vi "Sent.vi"(8 "error in (no error)":errorcluster, 11 "Mail in":refnum<class "Mail.lvclass">) -> (0 "error out":errorcluster, 3 "Mail out":refnum<class "Mail.lvclass">)   [LabVIEW 2023, in "HardwareAbstractionLayer_LVOOP.lvlib" / "Mail.lvclass"]
uses:
  Mail.lvclass
  Mail.lvclass/Mail.ctl
  <vilib>/smtpClient/LabVIEWSMTPClient.lvlib
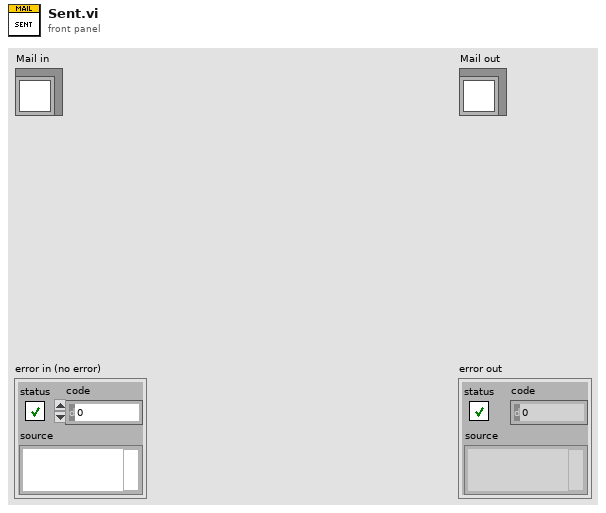
[diagram p1: front panel]
types:
  T1 = typedef "LabVIEWSMTPClient.lvlib/SmtpClientHandle.ctl" = refnum<k1>
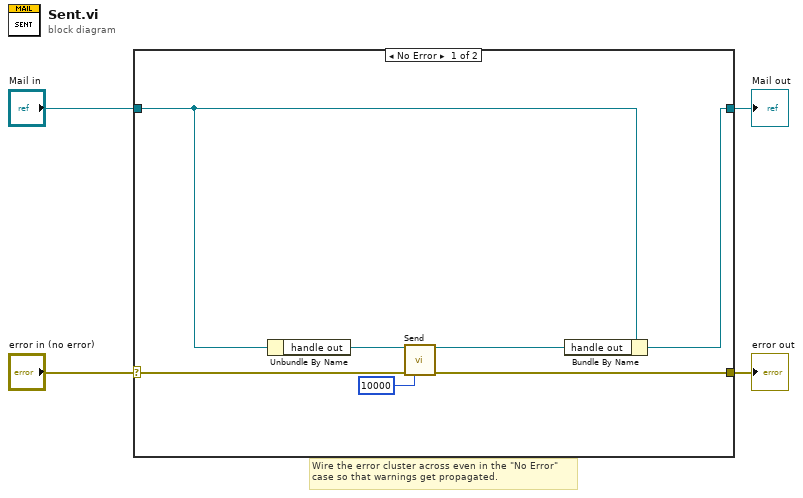
[diagram p0: block diagram]
diagram:
  # "Wire the error cluster across even in the \"No Error\"\ncase so that warnings get propagated."
  n1 = case shown="No Error" "error in (no error)" {
    selector: "error in (no error)" -> [w11 w13]
    tunnel: [w10 w13] -> w3
    tunnel: [w7 w12] -> w1
    tunnel: "Mail in" -> [w8 w12]
    frame No Error {
      n2 = Unbundle By Name(w8) -> ("handle out"=w9:T1)
      n3 = call <vilib>:"Send.vi"("handle in"=w9, "error in (no error)"=w11, "timeout in ms (10000)"=10000) -> ("handle out"=w6:T1, "error out"=w10:errorcluster)  [unwired: 10 in, 1 out]
      n4 = Bundle By Name(cluster=w8, "handle out"=w6) -> (w7:refnum<class "Mail.lvclass">)
    }
    frame Error {
    }
  }
  "error out" <- w3
  "Mail out" <- w1
